vi "Measurement UI.vi"() -> ()   [LabVIEW 2021, in "PWM Dimming UI.lvlib"]
uses:
  PWM Dimming UI.lvlib
panel:
  in  "MeasGraphs":T1(tab)
  out "Output VoltageV/STimeGraph":waveform(dbl)(graph)
  out "Output CurrentV/STimeGraph":waveform(dbl)(graph)
  out "PWMVoltageV/STimeGraph":waveform(dbl)(graph)
  out "Input VoltageV/STimeGraph":waveform(dbl)(graph)
  out "MeasTable":string[][](table)
  out "PWM Input V/S Output Duty Cycle":T2(graph)
  in  "AWG measure trigger":string
  out "Input duty cycle(%)":dbl[](array[numeric])
  out "Output duty cycle(%)":dbl[](array[numeric])
  out "PWM input voltage(scope amplitude)":dbl[](array[numeric])
  out "Scope dt":dbl
  out "SMU dt":dbl
  out "Input voltages(SMU)":dbl[](array[numeric])
  out "Output currents(SMU)":dbl[](array[numeric])
  out "Output voltages(SMU)":dbl[](array[numeric])
  in  "Load resource name":string
  in  "Source resource name":string
  in  "AWG resource name":string
  in  "Scope resource name":string
  in  "MeasConfigurations":T3(tab)=enum."Load Config"
  in  "Measurement timeout":dbl=10.0 caption="MEASUREMENT TIMEOUT" format="%.3ps"
  in  "Measurement timings":string="TIMINGS"
  in  "Duty cycle sweep type":string(combo)="Linear" caption="SWEEP TYPE"
  in  "Duty cycle single pulse/sweep pulse":bool=TRUE caption="DUTY CYCLE SINGLE PULSE/SWEEP PULSE"
  in  "Duty cycle config":string="DUTY CYCLE CONFIG"
  in  "Nominal output voltage":dbl=12.0 caption="NOMINAL OUTPUT VOLTAGE" format="%.3pV"
  in  "DUT setup time":dbl=1.0 caption="DUT SETUP TIME" format="%.3ps"
  in  "Duty cycle single point":dbl=50.0 caption="DUTY CYCLE" format="%.1f%"
  in  "Number of pulse cycle":i32=1 caption="NUMBER OF  PULSE CYCLES"
  in  "Start duty cycle":dbl=0.9 caption="START DUTY CYCLE" min=0.9 max=99.1 format="%.1f%"
  in  "Number of sweep points":i32=10 caption="NUMBER OF SWEEP POINTS"
  in  "Stop duty cycle":dbl=95.0 caption="STOP DUTY CYCLE" min=0.9 max=99.1 format="%.1p%"
  in  "PWM frequency":dbl=200.0 caption="FREQUENCY" format="%.3pHz"
  in  "Voltage compensation frequency":dbl(slide)=3530.0 caption="COMP. FREQUENCY" scale=50.0..1000000.0 scale format="%#_6pHz"
  in  "Voltage pole-zero ratio":dbl(slide)=2.0 caption="POLE-ZERO RATIO" scale=0.0625..16.0
  in  "Voltage gain bandwidth":dbl(slide)=2000.0 caption="GAIN BANDWIDTH" scale=10.0..1000000.0 scale format="%#_6pHz"
  in  "PPSResourceName":refnum<k15>="<Select Device>" caption="RESOURCE NAME"
  in  "Source transient response":i32(ring)=1038 caption="TRANSIENT RESPONSE" items=["Slow"=1041, "Normal"=1038, "Fast"=1039, "Custom"=1042]
  in  "Source sense":i32(ring)=1009 caption="SENSE" items=["Local"=1008, "Remote"=1009]
  in  "Source voltage level range":dbl=15.0 caption="VOLTAGE LEVEL RANGE" format="%#_6pV"
  in  "Source voltage level":dbl=12.0 caption="VOLTAGE LEVEL" format="%#_6pV"
  in  "Source current limit range":dbl=0.1 caption="CURRENT LIMIT RANGE" format="%#_6pA"
  in  "Source sourceadapt":string="Voltage SourceAdapt "
  in  "Current compensation frequency":dbl(slide)=250000.0 caption="COMP. FREQUENCY" scale=50.0..1000000.0 scale format="%#_6pHz"
  in  "Current pole-zero ratio":dbl(slide)=5.0 caption="POLE-ZERO RATIO" scale=0.0625..16.0
  in  "Current gain bandwidth":dbl(slide)=50000.0 caption="GAIN BANDWIDTH" scale=10.0..1000000.0 scale format="%#_6pHz"
  in  "Load current level range":dbl=0.1 caption="CURRENT LEVEL RANGE" format="%#_6pA"
  in  "Load sample rate":dbl=1800000.0 caption="SAMPLE RATE" format="%#_6pS/s"
  in  "Load pulse bias current level":dbl caption="PULSE BIAS CURRENT LEVEL" format="%#_6pA"
  in  "Load pulse current level":dbl=0.02 caption="PULSE CURRENT LEVEL" format="%#_6pA"
  in  "Load sourceadapt":string="Current SourceAdapt"
  in  "Load voltage limit range":dbl=15.0 caption="VOLTAGE LIMIT RANGE" format="%#_6pV"
  in  "Load sense":i32(ring)=1009 caption="SENSE" items=["Local"=1008, "Remote"=1009]
  in  "Load transient response":i32(ring)=1038 caption="TRANSIENT RESPONSE" items=["Slow"=1041, "Normal"=1038, "Fast"=1039, "Custom"=1042]
  in  "LoadResourceName":refnum<k15>="<Select Device>" caption="RESOURCE NAME"
  in  "AWGMeasureTrigger":tag caption="MEASURE TRIGGER"
  in  "AWG source trigger":string(combo)="PFI0" caption="SOURCE TRIGGER"
  in  "AWG triggers":string="Triggers"
  in  "AWG load impedence":dbl=100000.0 caption="LOAD IMPEDENCE" format="%#_pohm"
  in  "AWG dc offset":dbl=4.0 caption="DC OFFSET" format="%#_fV"
  in  "AWGResourceName":refnum<k15>="<Select Device>" caption="RESOURCE NAME"
  in  "AWG amplitude":dbl=8.0 caption="AMPLITUDE" format="%#_fV"
  in  "AWG channel name":string="0" caption="CHANNEL NAME"
  in  "Scope vertical range":dbl=15.0 caption="VERTICAL RANGE" format="%#_gV"
  in  "SCOPEResourceName":refnum<k15>="<Select Device>" caption="RESOURCE NAME"
  in  "Scope probe attenuation":dbl=10.0 caption="PROBE ATTENUATION" format="%#_6p"
  in  "Scope sample rate":dbl=1800000.0 caption="SAMPLE RATE" format="%#_6pS/s"
  in  "Scope input channel name":string="0" caption="INPUT CHANNEL NAME"
  in  "Scope vertical coupling":enum32{"AC", "DC"}(ring)=enum."DC" caption="VERTICAL COUPLING"
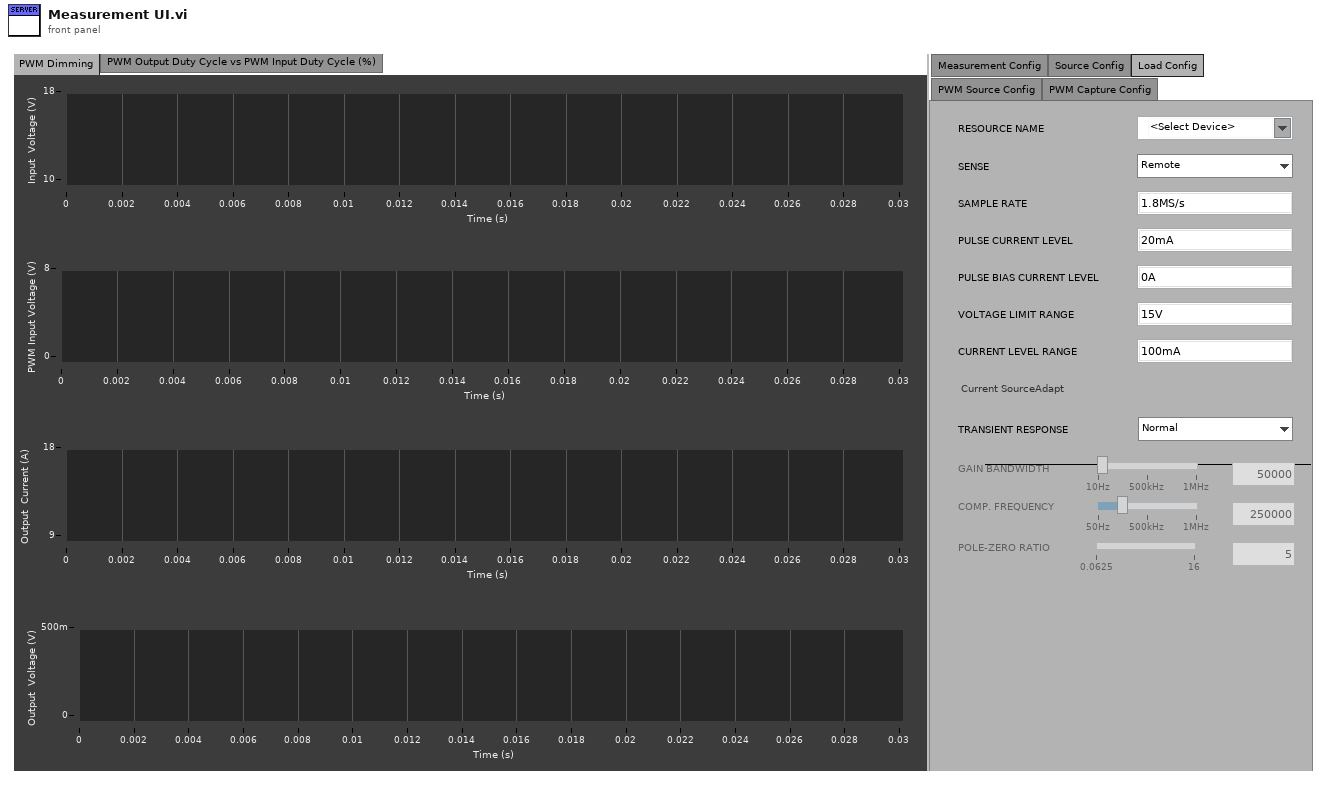
[diagram p1: front panel]
types:
  T1 = enum32{"PWM Dimming", "PWM Output Duty Cycle vs PWM Input Duty Cycle (%)", "Hidden Controls"}
  T2 = cluster{"Source voltages":dbl[], "Load voltages":dbl[]}
  T3 = enum32{"Measurement Config", "Source Config", "Load Config", "PWM Source Config", "PWM Capture Config"}
  T4 = enum8{"Enabled", "Disabled", "Disabled and Grayed Out"}
  T5 = cluster{"Output duty cycle(%)":dbl[], "Input duty cycle(%)":dbl[]}
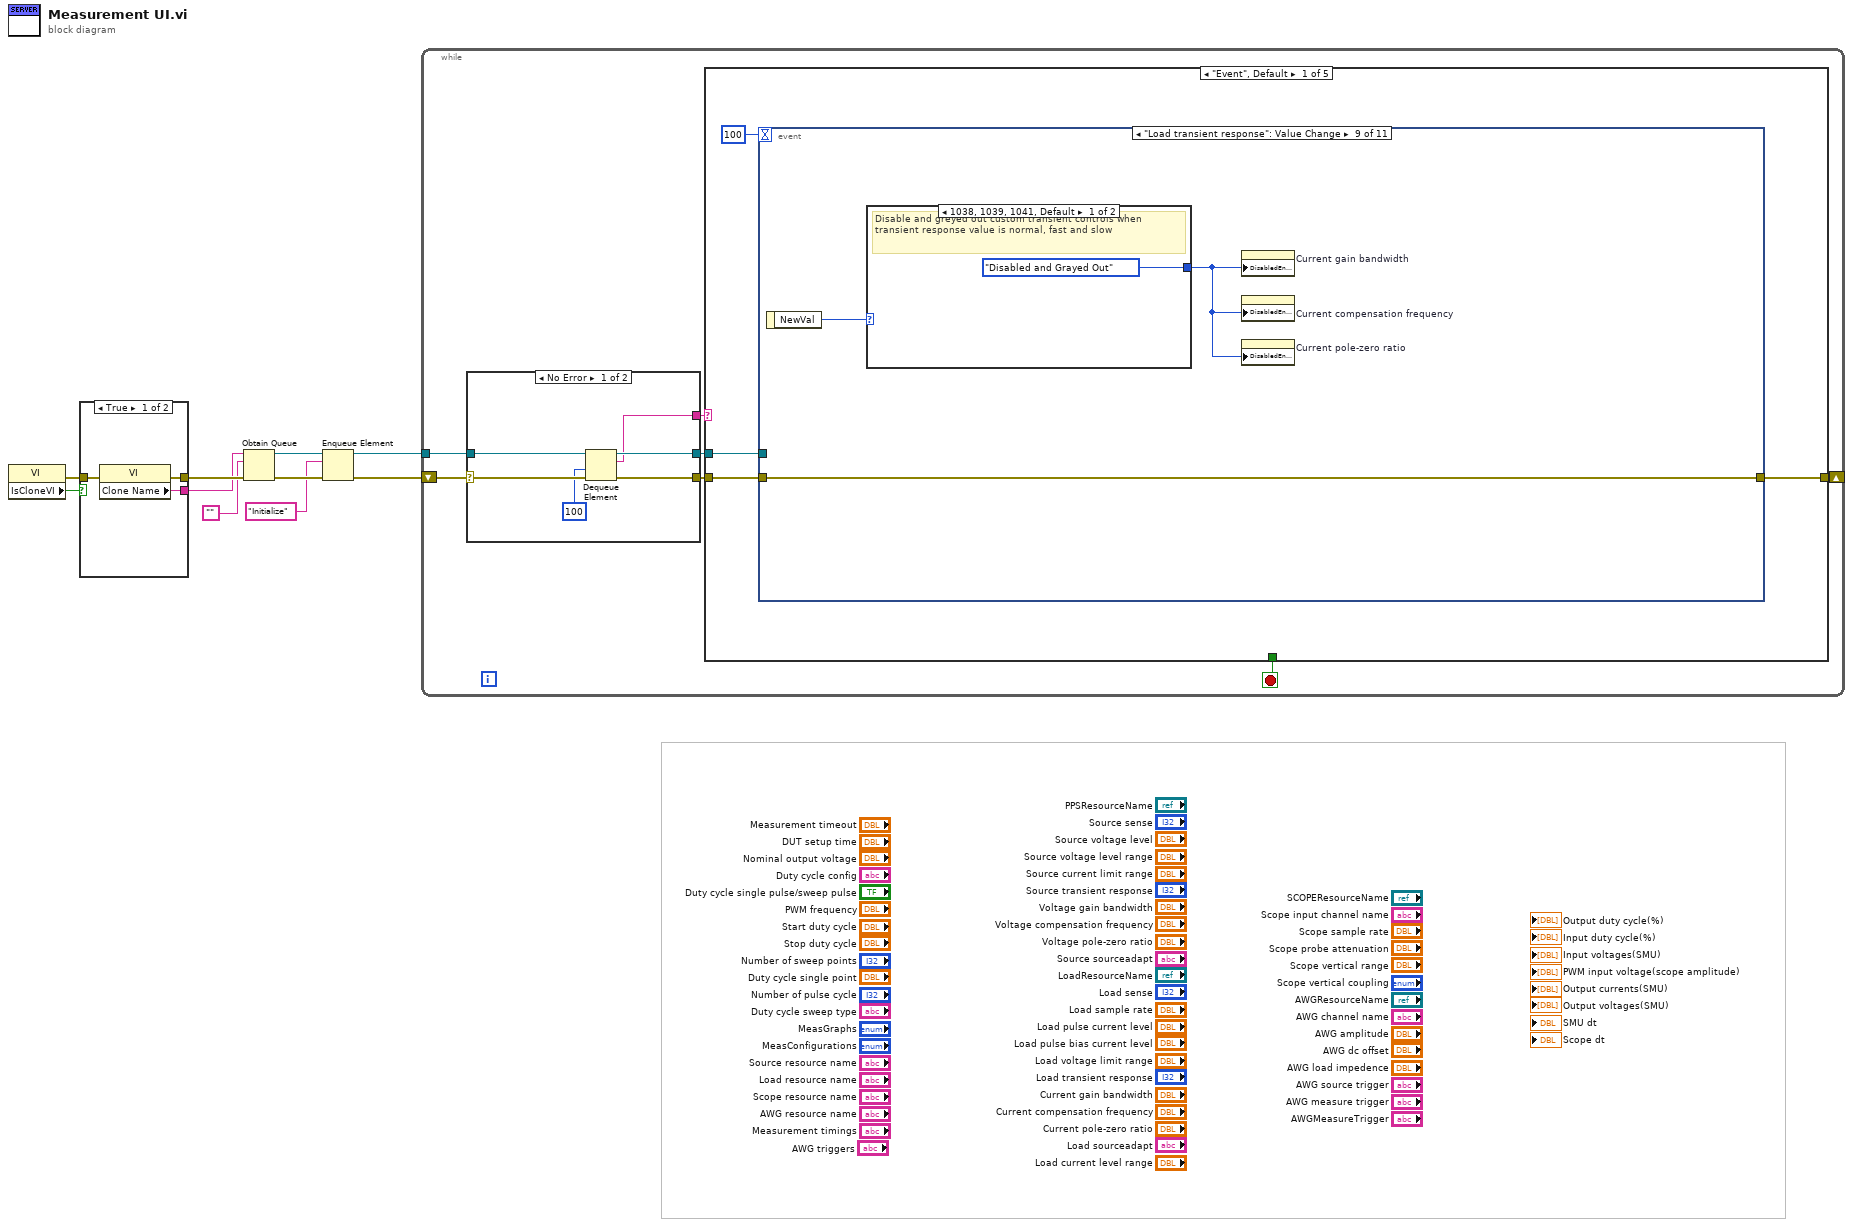
[diagram p0: block diagram]
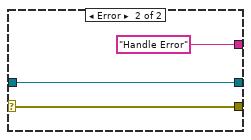
[diagram p2: hidden frame]
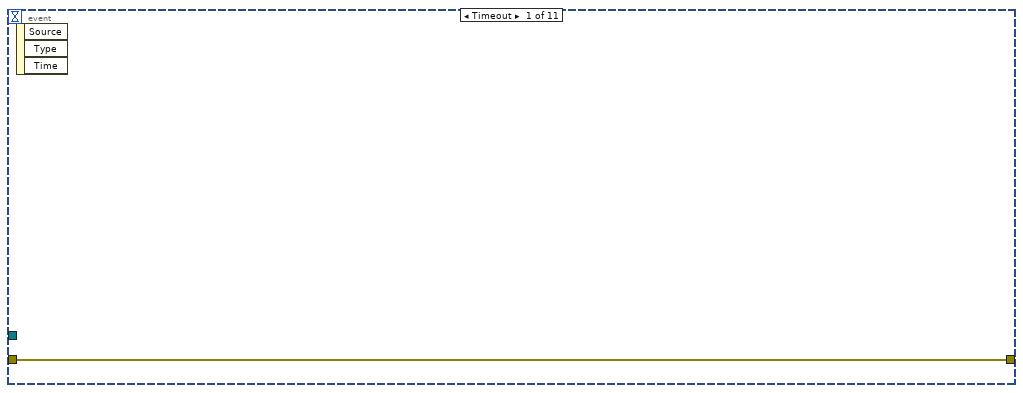
[diagram p3: hidden frame]
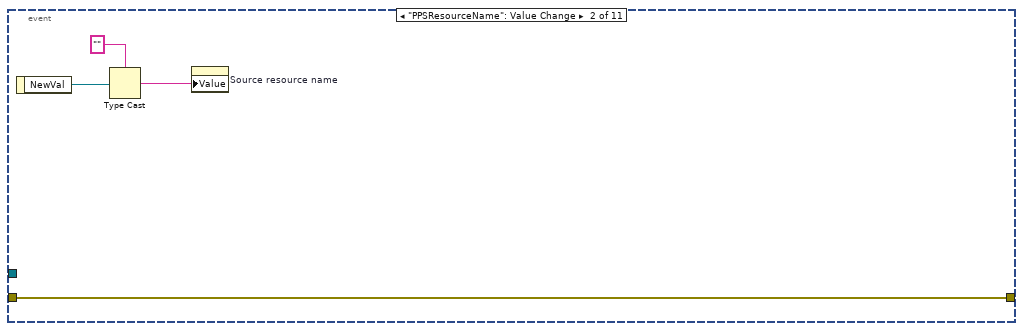
[diagram p4: hidden frame]
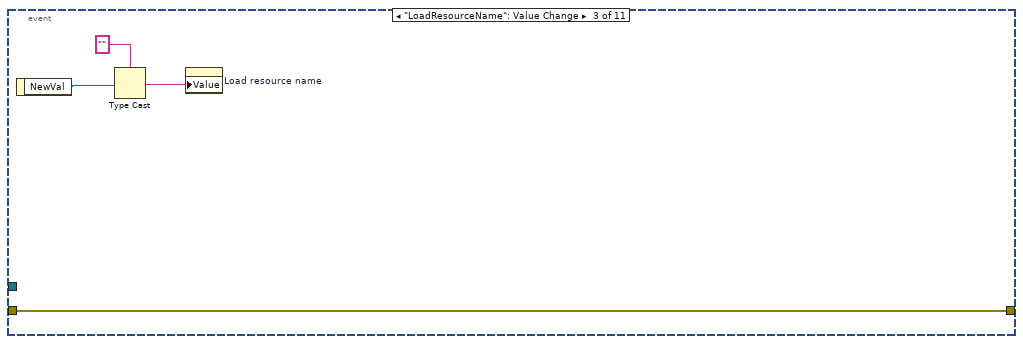
[diagram p5: hidden frame]
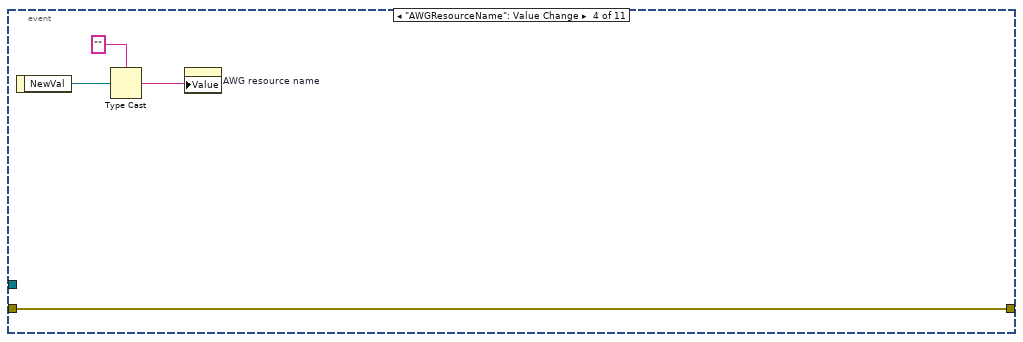
[diagram p6: hidden frame]
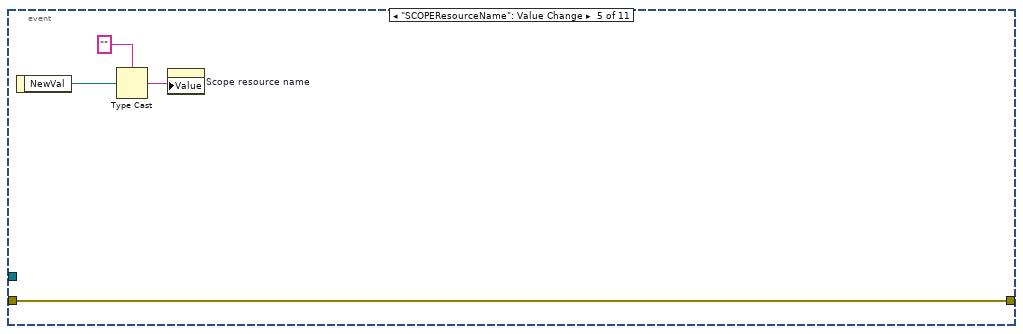
[diagram p7: hidden frame]
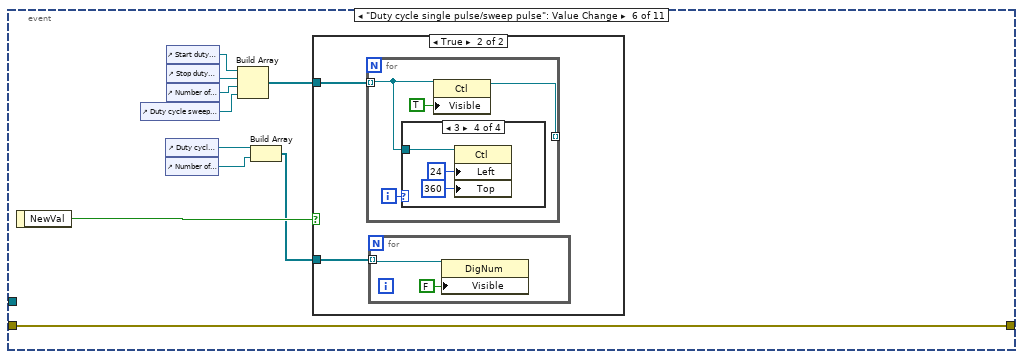
[diagram p8: hidden frame]
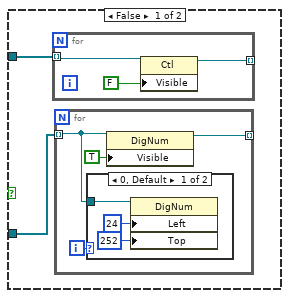
[diagram p9: hidden frame]
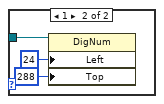
[diagram p10: hidden frame]
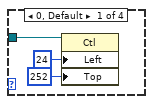
[diagram p11: hidden frame]
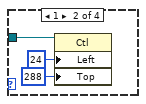
[diagram p12: hidden frame]
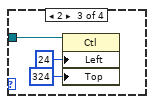
[diagram p13: hidden frame]
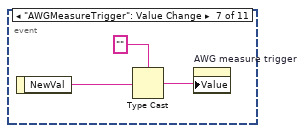
[diagram p14: hidden frame]
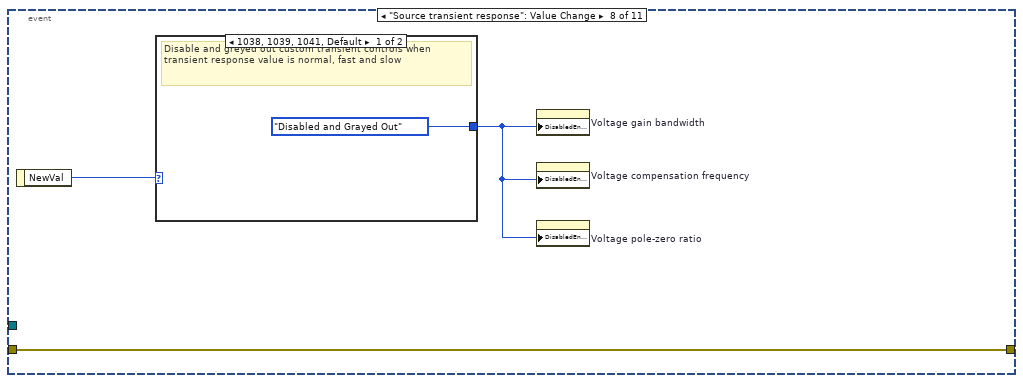
[diagram p15: hidden frame]
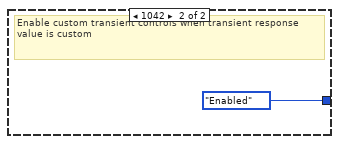
[diagram p16: hidden frame]
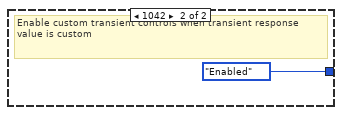
[diagram p17: hidden frame]
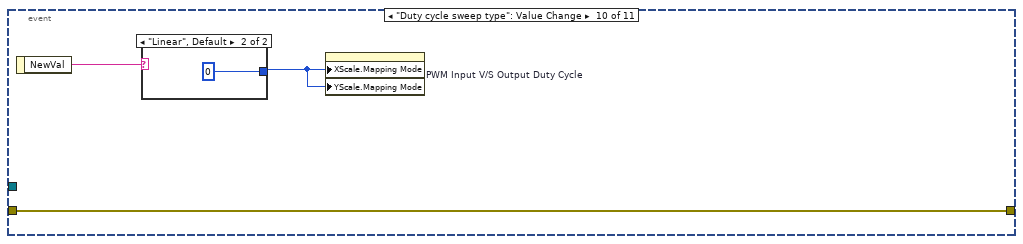
[diagram p18: hidden frame]
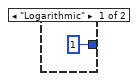
[diagram p19: hidden frame]
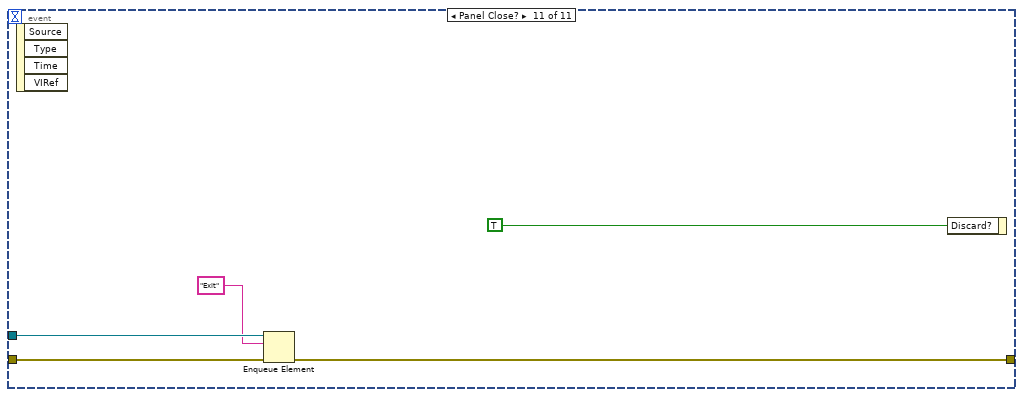
[diagram p20: hidden frame]
diagram:
  n1 = property class="VI"() -> (error out=w1:errorcluster, "IsCloneVI"=w2:bool)  [unwired: 2 in, 1 out]
  n2 = case shown="True" w2 {
    tunnel: [w13 w16] -> w10
    tunnel: [w12 w15] -> w9
    tunnel: w1 -> [w11 w14]
    frame True {
      n3 = property class="VI"(error in=w11) -> (error out=w13:errorcluster, "Clone Name"=w12:string)  [unwired: 1 in, 1 out]
    }
    frame False {
      n4 = property class="VI"(error in=w14) -> (error out=w16:errorcluster, "Name"=w15:string)  [unwired: 1 in, 1 out]
    }
  }
  n5 = Obtain Queue(name (unnamed)=w9, element data type="", error in (no error)=w10) -> (queue out=w6:refnum<queue>, error out=w8:errorcluster)  [unwired: 2 in, 1 out]
  n6 = Enqueue Element(queue=w6, element="Initialize", error in (no error)=w8) -> (queue out=w5:refnum<queue>, error out=w7:errorcluster)  [unwired: 1 in, 1 out]
  n7 = while {
    shift-right: [w18] -> _
    shift-left: w7 -> [w23]
    tunnel: w5 -> [w21]
    stop <- w17 stop-if-true
    n8 = case shown="No Error" w23 {
      selector: w23 -> [w29 w32]
      tunnel: [w28 w32] -> w22
      tunnel: w21 -> [w27 w31]
      tunnel: [w26 w31] -> w20
      tunnel: [w25 "Handle Error"] -> w19
      frame No Error {
        n9 = Dequeue Element(queue=w27, timeout in ms (-1)=100, error in (no error)=w29) -> (queue out=w26:refnum<queue>, element=w25:string, error out=w28:errorcluster)  [unwired: 1 out]
      }
      frame Error {
      }
    }
    n10 = case shown="\"Event\", Default" w19 {
      tunnel: w22 -> [w35 w131 w142 w172 w173]
      tunnel: w20 -> [w33 _ _ w170 _]
      tunnel: [w36 w131 w141 w167 w173] -> w18
      tunnel: [_ FALSE _ TRUE _] -> w17
      frame "Event", Default {
        n11 = event shown="[8] \"Load transient response\": Value Change" {
          selector: _ -> [_ _ _ _ _ _ _ _ _ _ _]
          dyn-events: _ -> [_ _ _ _ _ _ _ _ _ _ _]
          timeout: 100 -> [_ _ _ _ _ _ _ _ _ _ _]
          tunnel: [w37 w38 w42 w46 w50 w62 _ w103 w108 w113 w119] -> w36
          tunnel: w35 -> [w37 w38 w42 w46 w50 w62 _ w103 w108 w113 w120]
          tunnel: w33 -> [_ _ _ _ _ _ _ _ _ _ w118]
          event Timeout {
            n12 = event-data() -> ()  [unwired: 1 in, 3 out]
          }
          event "PPSResourceName": Value Change {
            n13 = event-data() -> ("NewVal"=w40:refnum<k15>)  [unwired: 1 in]
            n14 = Type Cast(type="", x=w40) -> (*(type *) &x=w39:string)
            n15 = property on="Source resource name" class="Str"("Value"=w39) -> ()  [unwired: 2 in, 2 out]
          }
          event "LoadResourceName": Value Change {
            n16 = event-data() -> ("NewVal"=w44:refnum<k15>)  [unwired: 1 in]
            n17 = Type Cast(type="", x=w44) -> (*(type *) &x=w43:string)
            n18 = property on="Load resource name" class="Str"("Value"=w43) -> ()  [unwired: 2 in, 2 out]
          }
          event "AWGResourceName": Value Change {
            n19 = event-data() -> ("NewVal"=w48:refnum<k15>)  [unwired: 1 in]
            n20 = Type Cast(type="", x=w48) -> (*(type *) &x=w47:string)
            n21 = property on="AWG resource name" class="Str"("Value"=w47) -> ()  [unwired: 2 in, 2 out]
          }
          event "SCOPEResourceName": Value Change {
            n22 = event-data() -> ("NewVal"=w52:refnum<k15>)  [unwired: 1 in]
            n23 = Type Cast(type="", x=w52) -> (*(type *) &x=w51:string)
            n24 = property on="Scope resource name" class="Str"("Value"=w51) -> ()  [unwired: 2 in, 2 out]
          }
          event "Duty cycle single pulse/sweep pulse": Value Change {
            n25 = event-data() -> ("NewVal"=w63:bool)  [unwired: 1 in]
            n26 = control-ref of="Duty cycle sweep type"() -> (w58:refnum<vi>)
            n27 = control-ref of="Duty cycle single point"() -> (w56:refnum<vi>)
            n28 = control-ref of="Number of pulse cycle"() -> (w55:refnum<vi>)
            n29 = control-ref of="Start duty cycle"() -> (w61:refnum<vi>)
            n30 = control-ref of="Stop duty cycle"() -> (w60:refnum<vi>)
            n31 = control-ref of="Number of sweep points"() -> (w59:refnum<vi>)
            n32 = Build Array(w61, w60, w59, w58) -> (w57:refnum<vi>[])
            n33 = Build Array(w56, w55) -> (w54:refnum<vi>[])
            n34 = case shown="True" w63 {
              tunnel: w57 -> [w65 w80]
              tunnel: w54 -> [w64 w79]
              frame False {
                n35 = for {
                  tunnel: w65 -> [w77] mode=indexing
                  tunnel: [w76] -> _ mode=indexing
                  n36 = property class="Ctl"(reference=w77, "Visible"=FALSE) -> (reference out=w76:refnum<vi>)  [unwired: 1 in, 1 out]
                }
                n37 = for {
                  tunnel: w64 -> [w67] mode=indexing
                  tunnel: [w66] -> _ mode=indexing
                  i -> [w68]
                  n38 = case shown="0, Default" w68 {
                    tunnel: w67 -> [w72 w73]
                    frame 0, Default {
                      n39 = property class="DigNum"(reference=w72, "Left"=24 ("Position:Left"), "Top"=252 ("Position:Top")) -> ()  [unwired: 1 in, 2 out]
                    }
                    frame 1 {
                      n40 = property class="DigNum"(reference=w73, "Left"=24 ("Position:Left"), "Top"=288 ("Position:Top")) -> ()  [unwired: 1 in, 2 out]
                    }
                  }
                  n41 = property class="DigNum"(reference=w67, "Visible"=TRUE) -> (reference out=w66:refnum<vi>)  [unwired: 1 in, 1 out]
                }
              }
              frame True {
                n42 = for {
                  tunnel: w80 -> [w83] mode=indexing
                  tunnel: [w85] -> _ mode=indexing
                  i -> [w84]
                  n43 = case shown="3" w84 {
                    tunnel: w83 -> [w89 w92 w93 w96]
                    frame 0, Default {
                      n44 = property class="Ctl"(reference=w89, "Left"=24 ("Position:Left"), "Top"=252 ("Position:Top")) -> ()  [unwired: 1 in, 2 out]
                    }
                    frame 1 {
                      n45 = property class="Ctl"(reference=w92, "Left"=24 ("Position:Left"), "Top"=288 ("Position:Top")) -> ()  [unwired: 1 in, 2 out]
                    }
                    frame 2 {
                      n46 = property class="Ctl"(reference=w93, "Left"=24 ("Position:Left"), "Top"=324 ("Position:Top")) -> ()  [unwired: 1 in, 2 out]
                    }
                    frame 3 {
                      n47 = property class="Ctl"(reference=w96, "Left"=24 ("Position:Left"), "Top"=360 ("Position:Top")) -> ()  [unwired: 1 in, 2 out]
                    }
                  }
                  n48 = property class="Ctl"(reference=w83, "Visible"=TRUE) -> (reference out=w85:refnum<vi>)  [unwired: 1 in, 1 out]
                }
                n49 = for {
                  tunnel: w79 -> [w81] mode=indexing
                  n50 = property class="DigNum"(reference=w81, "Visible"=FALSE) -> ()  [unwired: 1 in, 2 out]
                }
              }
            }
          }
          event "AWGMeasureTrigger": Value Change {
            n51 = event-data() -> ("NewVal"=w100:tag)  [unwired: 1 in]
            n52 = Type Cast(type="", x=w100) -> (*(type *) &x=w99:string)
            n53 = property on="AWG measure trigger" class="Str"("Value"=w99) -> ()  [unwired: 2 in, 2 out]
          }
          event "Source transient response": Value Change {
            n54 = event-data() -> ("NewVal"=w104:i32)  [unwired: 1 in]
            n55 = case shown="1038, 1039, 1041, Default" w104 {
              tunnel: [T4."Disabled and Grayed Out" ("Disabled") T4."Enabled" ("Disabled")] -> w102
              frame 1038, 1039, 1041, Default {
                # "Disable and greyed out custom transient controls when transient response value is normal, fast and slow"
              }
              frame 1042 {
                # "Enable custom transient controls when transient response value is custom"
              }
            }
            n56 = property on="Voltage gain bandwidth" class="Slide (strict)"("DisabledEnum"=w102) -> ()  [unwired: 2 in, 2 out]
            n57 = property on="Voltage compensation frequency" class="Slide (strict)"("DisabledEnum"=w102) -> ()  [unwired: 2 in, 2 out]
            n58 = property on="Voltage pole-zero ratio" class="Slide (strict)"("DisabledEnum"=w102) -> ()  [unwired: 2 in, 2 out]
          }
          event "Load transient response": Value Change {
            n59 = event-data() -> ("NewVal"=w109:i32)  [unwired: 1 in]
            n60 = case shown="1038, 1039, 1041, Default" w109 {
              tunnel: [T4."Disabled and Grayed Out" ("Disabled") T4."Enabled" ("Disabled")] -> w107
              frame 1038, 1039, 1041, Default {
                # "Disable and greyed out custom transient controls when transient response value is normal, fast and slow"
              }
              frame 1042 {
                # "Enable custom transient controls when transient response value is custom"
              }
            }
            n61 = property on="Current gain bandwidth" class="Slide (strict)"("DisabledEnum"=w107) -> ()  [unwired: 2 in, 2 out]
            n62 = property on="Current compensation frequency" class="Slide (strict)"("DisabledEnum"=w107) -> ()  [unwired: 2 in, 2 out]
            n63 = property on="Current pole-zero ratio" class="Slide (strict)"("DisabledEnum"=w107) -> ()  [unwired: 2 in, 2 out]
          }
          event "Duty cycle sweep type": Value Change {
            n64 = event-data() -> ("NewVal"=w114:string)  [unwired: 1 in]
            n65 = case shown="\"Linear\", Default" w114 {
              tunnel: [u8 1 ("X Scale.Mapping Mode") u8 0 ("X Scale.Mapping Mode")] -> w112
              frame "Logarithmic" {
              }
              frame "Linear", Default {
              }
            }
            n66 = property on="PWM Input V/S Output Duty Cycle" class="XYGraph (strict)"("XScale.Mapping Mode"=w112, "YScale.Mapping Mode"=w112) -> ()  [unwired: 2 in, 2 out]
          }
          event Panel Close? {
            n67 = event-data() -> ()  [unwired: 1 in, 4 out]
            n68 = Enqueue Element(queue=w118, element="Exit", error in (no error)=w120) -> (error out=w119:errorcluster)  [unwired: 1 in, 2 out]
            n69 = event-data("Discard?"=TRUE) -> ()  [unwired: 1 in, 1 out]
          }
        }
      }
      frame "Initialize" {
        w122 = T4."Disabled and Grayed Out" ("Disabled")
        w123 = T4."Disabled and Grayed Out" ("Disabled")
        n70 = control-ref of="SCOPEResourceName"() -> (w125:refnum<vi>)
        n71 = control-ref of="AWGResourceName"() -> (w124:refnum<vi>)
        n72 = control-ref of="PPSResourceName"() -> (w127:refnum<vi>)
        n73 = control-ref of="LoadResourceName"() -> (w126:refnum<vi>)
        n74 = property on="Current gain bandwidth" class="Slide (strict)"("DisabledEnum"=w123) -> ()  [unwired: 2 in, 2 out]
        n75 = property on="Current compensation frequency" class="Slide (strict)"("DisabledEnum"=w123) -> ()  [unwired: 2 in, 2 out]
        n76 = property on="Current pole-zero ratio" class="Slide (strict)"("DisabledEnum"=w123) -> ()  [unwired: 2 in, 2 out]
        n77 = Build Array(w127, w126, w125, w124) -> (w129:refnum<vi>[])
        n78 = for {
          tunnel: w129 -> [w132] mode=indexing
          tunnel: "<Select Device>" -> [w135]
          n79 = Type Cast(type=refnum<k15> refnum ("Value"), x=w135) -> (*(type *) &x=w133:refnum<k15>)
          n80 = property class="IVIName"(reference=w132, "Value"=w133) -> ()  [unwired: 1 in, 2 out]
        }
        n81 = property on="Voltage gain bandwidth" class="Slide (strict)"("DisabledEnum"=w122) -> ()  [unwired: 2 in, 2 out]
        n82 = property on="Voltage compensation frequency" class="Slide (strict)"("DisabledEnum"=w122) -> ()  [unwired: 2 in, 2 out]
        n83 = property on="Voltage pole-zero ratio" class="Slide (strict)"("DisabledEnum"=w122) -> ()  [unwired: 2 in, 2 out]
      }
      frame "Post UI Update" {
        # "This case will be triggered, after framework updates the User interface with result values."
        n84 = local read "PWM input voltage(scope amplitude)"() -> (w145:dbl[])
        n85 = local read "Output voltages(SMU)"() -> (w150:dbl[])
        n86 = local read "Output currents(SMU)"() -> (w151:dbl[])
        n87 = local read "Output duty cycle(%)"() -> (w155:dbl[])
        n88 = local read "Input voltages(SMU)"() -> (w152:dbl[])
        n89 = local read "Input duty cycle(%)"() -> (w154:dbl[])
        n90 = property on="Duty cycle sweep type" class="CmbBox"() -> ("Value"=w140:string)  [unwired: 2 in, 2 out]
        n91 = local read "Scope dt"() -> (w144:dbl)
        n92 = local read "SMU dt"() -> (w149:dbl)
        n93 = case shown="\"Linear\", Default" w140 {
          tunnel: [u8 1 ("X Scale.Mapping Mode") u8 0 ("X Scale.Mapping Mode")] -> w136
          frame "Logarithmic" {
          }
          frame "Linear", Default {
          }
        }
        n94 = Bundle By Name("Y"=w152, "dt"=w149) -> (→"Input VoltageV/STimeGraph":waveform(dbl))  [unwired: 1 in]
        n95 = Bundle By Name("Y"=w151, "dt"=w149) -> (→"Output CurrentV/STimeGraph":waveform(dbl))  [unwired: 1 in]
        n96 = Bundle By Name("Y"=w150, "dt"=w149) -> (→"Output VoltageV/STimeGraph":waveform(dbl))  [unwired: 1 in]
        n97 = Bundle By Name("Y"=w145, "dt"=w144) -> (→"PWMVoltageV/STimeGraph":waveform(dbl))  [unwired: 1 in]
        n98 = control-ref of="PWM Input V/S Output Duty Cycle"() -> (w143:refnum<vi>)
        n99 = Bundle("Output duty cycle(%)"=w155, "Input duty cycle(%)"=w154) -> (→"PWM Input V/S Output Duty Cycle":T5)  [unwired: 1 in]
        n100 = local read "Output duty cycle(%)"() -> (w138:dbl[])
        n101 = property class="XYGraph (strict)"(reference=w143, error in=w142, "XScale.Mapping Mode"=w136, "YScale.Mapping Mode"=w136) -> (error out=w141:errorcluster)  [unwired: 1 out]
        n102 = local read "Input duty cycle(%)"() -> (w139:dbl[])
        n103 = for {
          tunnel: w139 -> [w159] mode=indexing
          tunnel: w138 -> [w158] mode=indexing
          tunnel: [w157] -> w137 mode=indexing
          w162 = "%.3f" ("initial string")
          n104 = Format Into String(format string=w162, w159) -> (resulting string=w161:string)  [unwired: 2 in, 1 out]
          n105 = Format Into String(format string=w162, initial string="|   ", w158) -> (resulting string=w160:string)  [unwired: 1 in, 1 out]
          n106 = Build Array(w161, w160) -> (w157:string[])
        }
        "MeasTable" <- w137
      }
      frame "Exit" {
        # "This case is triggered to close the User Interface from framework"
        n107 = Flush Queue(queue=w170, error in (no error)=w172) -> (queue out=w169:refnum<queue>, error out=w168:errorcluster)  [unwired: 1 out]
        n108 = Release Queue(queue=w169, force destroy? (F)=TRUE, error in (no error)=w168) -> (error out=w167:errorcluster)  [unwired: 2 out]
      }
      frame "Handle Error" {
      }
    }
  }
